vi "Test_Status.vi"() -> ()   [LabVIEW 2016]
panel:
  out "Test Status":string
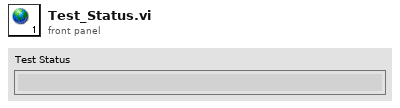
[diagram p1: front panel]
diagram:
